vi "set_frequency.vi"(8 "error in (no error)":errorcluster, 10 "Frequency":dbl, 11 "Keysight 33511B in":refnum<class "Keysight 33511B.lvclass">) -> (0 "error out":errorcluster, 3 "Keysight 33511B out":refnum<class "Keysight 33511B.lvclass">)   [LabVIEW 2020, in "Keysight 33511B.lvclass"]
uses:
  Keysight 33511B.lvclass
  Keysight 33511B.lvclass/Keysight 33511B.ctl
  Function Generator/Function Generator.lvclass
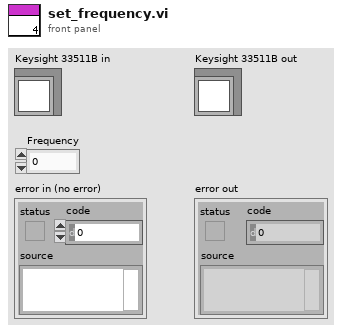
[diagram p1: front panel]
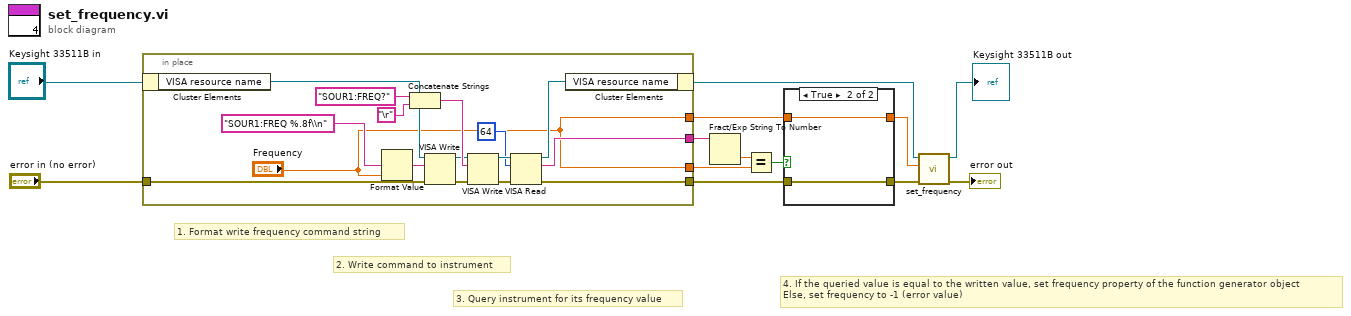
[diagram p0: block diagram]
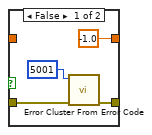
[diagram p2: hidden frame]
diagram:
  # "4. If the queried value is equal to the written value, set frequency property of the function generator object\nElse, set frequency to -1 (error value)"
  # "3. Query instrument for its frequency value"
  # "2. Write command to instrument"
  # "1. Format write frequency command string"
  n1 = in-place {
    in-place-border: "error in (no error)" -> [w19]
    in-place-border: ["Frequency"] -> w9
    in-place-border: [w18] -> w8
    in-place-border: ["Frequency"] -> w7
    in-place-border: [w17] -> w6
    n2 = in-place-cluster #1("Keysight 33511B in") -> ("VISA resource name"=w15:refnum<visa-resource-name>)
    n3 = Format Value(format string="SOUR1:FREQ %.8f\\n", value (0)="Frequency") -> (output string=w24:string)  [unwired: 1 in]
    n4 = Concatenate Strings("SOUR1:FREQ?", "\r") -> (w27:string)
    n5 = VISA Write(VISA resource name=w15, write buffer=w24, error in (no error)=w19) -> (VISA resource name out=w25:refnum<visa-resource-name>, error out=w26:errorcluster)  [unwired: 1 out]
    n6 = VISA Write(VISA resource name=w25, write buffer=w27, error in (no error)=w26) -> (VISA resource name out=w28:refnum<visa-resource-name>, error out=w29:errorcluster)  [unwired: 1 out]
    n7 = VISA Read(VISA resource name=w28, byte count=u32 64, error in (no error)=w29) -> (VISA resource name out=w16:refnum<visa-resource-name>, read buffer=w17:string, error out=w18:errorcluster)  [unwired: 1 out]
    n8 = in-place-cluster #1("VISA resource name"=w16) -> (w5:refnum<class "Keysight 33511B.lvclass">)
  }
  n9 = Fract/Exp String To Number(string=w6) -> (number=w13:dbl)  [unwired: 3 in, 1 out]
  n10 = Equal?(x=w13, y=w7) -> (x = y?=w12:bool)
  n11 = case shown="True" w12 {
    tunnel: w9 -> [_ w35]
    tunnel: w8 -> [w31 w34]
    tunnel: [-1.0 w35] -> w10
    tunnel: [w30 w34] -> w11
    frame False {
      n12 = call <vilib>:"Error Cluster From Error Code.vi"("error in (no error)"=w31, "error code (0)"=5001) -> ("error out"=w30:errorcluster)  [unwired: 7 in]
    }
    frame True {
    }
  }
  n13 = call-parent "set_frequency.vi"("error in (no error)"=w11, "Frequency"=w10, "Function Generator in"=w5) -> ("error out"=→"error out":errorcluster, "Function Generator out"=→"Keysight 33511B out":refnum<class "Keysight 33511B.lvclass">)  [unwired: 7 in]
